vi "Start.vi"(8 "error in (no error)":errorcluster, 11 "TCPMessaging in":refnum<class "TCPMessaging.lvclass">) -> (0 "error out":errorcluster, 3 "TCPMessaging out":refnum<class "TCPMessaging.lvclass">)   [LabVIEW 2020, in "Vecto.lvlib" / "TCPMessaging.lvclass"]
uses:
  TCPMessaging.lvclass
  TCPMessaging.lvclass/TCPMessaging.ctl
  Client Loops.vi
  Server Loops.vi
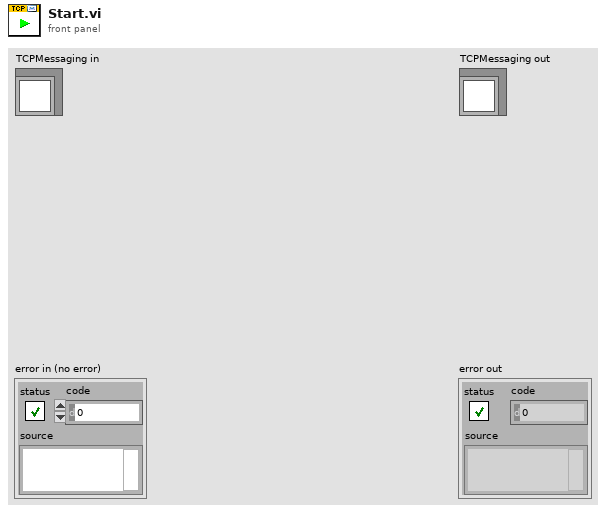
[diagram p1: front panel]
types:
  T1 = typedef "Vecto.lvlib/TCPMessaging.lvclass/TCP Mode.ctl" = enum16{"Client", "Server"}
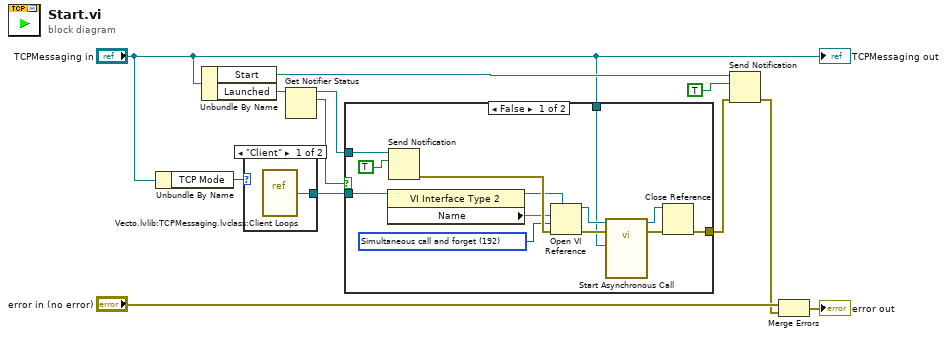
[diagram p0: block diagram]
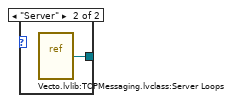
[diagram p3: hidden frame]
diagram:
  n1 = Unbundle By Name("TCPMessaging in") -> ("TCP Mode"=w11:T1)
  n2 = Unbundle By Name("TCPMessaging in") -> ("Start"=w5:refnum<notifier>, "Launched"=w8:refnum<notifier>)
  n3 = case shown="\"Client\"" w11 {
    tunnel: [w13 w14] -> w9
    frame "Client" {
      n4 = vi-ref "Vecto.lvlib:TCPMessaging.lvclass:Client Loops.vi"() -> (w13:refnum<vi>)
    }
    frame "Server" {
      n5 = vi-ref "Vecto.lvlib:TCPMessaging.lvclass:Server Loops.vi"() -> (w14:refnum<vi>)
    }
  }
  n6 = Get Notifier Status(notifier=w8) -> (notifier out=w6:refnum<notifier>, current notification=w7:bool)  [unwired: 1 in, 3 out]
  n7 = case shown="False" w7 {
    tunnel: w9 -> [w19 _]
    tunnel: w6 -> [w18 _]
    tunnel: [w16 _] -> w4
    tunnel: "TCPMessaging in" -> [w15 _]
    frame False {
      w20 = 192 items=["Record modifications"=1, "Open templates for editing"=2, "Prompt user to save"=4, "Prepare for reentrant run"=8, "Prompt to find missing subVIs"=16, "Hide loading dialog box"=32, "Enable simultaneous calls"=64, "Prepare to call and forget"=128, "Simultaneous call and forget"=192, "Prepare to call and collect"=256, "Simultaneous call and collect"=320]
      n8 = property class="VI Interface Type 2"(reference=w19) -> (reference out=w22:refnum<vi>, "Name"=w21:string)  [unwired: 1 in, 1 out]
      n9 = Send Notification(notification=TRUE, notifier=w18) -> (error out=w27:errorcluster)  [unwired: 1 in, 1 out]
      n10 = Open VI Reference(type specifier VI Refnum (for type only)=w22, vi path=w21, options=w20, error in (no error)=w27) -> (vi reference=w24:refnum<vi>, error out=w23:errorcluster)  [unwired: 2 in]
      n11 = call-by-ref "Start Asynchronous Call"(reference=w24, error in=w23, "TCPMessaging in"=w15) -> (reference out=w26:refnum<vi>, error out=w25:errorcluster)  [unwired: 11 in]
      n12 = Close Reference(reference=w26, error in (no error)=w25) -> (error out=w16:errorcluster)
    }
    frame True {
    }
  }
  n13 = Send Notification(notification=TRUE, notifier=w5, error in (no error)=w4) -> (error out=w2:errorcluster)  [unwired: 1 out]
  n14 = Merge Errors("error in (no error)", w2) -> (→"error out":errorcluster)
  "TCPMessaging out" <- "TCPMessaging in"
